vi "forceToVoltage.vi"(8 "error in (no error)":errorcluster, 9 "Pressure Servo Settings":T1={"Center Point"=2.5, "Area"=0.004536, "PA to PSI"=0.000145038, "Off Value"=0.004536} {"Off Value" format="%.3f"; "PA to PSI" format="%.9f"; "Area" format="%.9f"; "Center Point" format="%.3f"}, 10 "Force":dbl[unit], 11 "Force To Pressure Servo Valve Voltage in":refnum<class "Force To Pressure Servo Valve Voltage.lvclass">) -> (0 "error out":errorcluster, 1 "Voltage 2":dbl[unit], 2 "Voltage 1":dbl[unit], 3 "Force To Pressure Servo Valve Voltage out":refnum<class "Force To Pressure Servo Valve Voltage.lvclass">)   [LabVIEW 2015, in "Force To Pressure Servo Valve Voltage.lvclass"]
uses:
  Force To Pressure Servo Valve Voltage.lvclass
  Typedefs/Pressure Servo Valve Settings.ctl
  Typedefs/FAMT Typedefs.lvlib
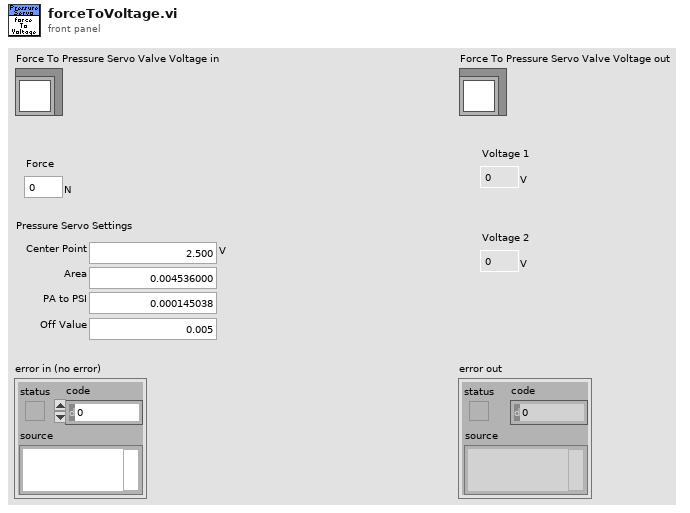
[diagram p1: front panel]
types:
  T1 = typedef "FAMT Typedefs.lvlib/Pressure Servo Valve Settings.ctl" = cluster{"Center Point":dbl[unit], "Area":dbl, "PA to PSI":dbl, "Off Value":dbl}
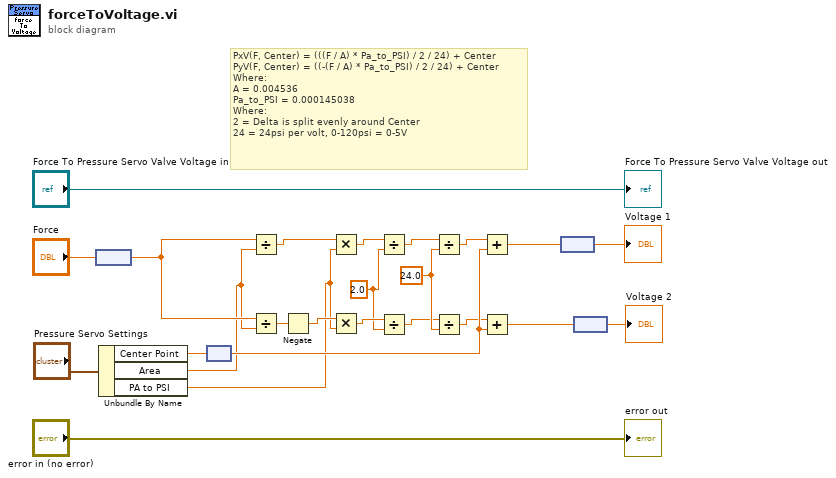
[diagram p0: block diagram]
diagram:
  w15 = 24.0 ("y")
  w19 = 2.0 ("y")
  # "PxV(F, Center) = (((F / A) * Pa_to_PSI) / 2 / 24) + Center\nPyV(F, Center) = ((-(F / A) * Pa_to_PSI) / 2 / 24) + Center\nWhere:\nA = 0.004536\nPa_to_PSI = 0.000145038\nWhere:\n2 = Delta is split evenly around Center\n24 = 24psi per volt, 0-120psi = 0-5V"
  n1 = node("Force") -> (w17:dbl)
  n2 = Unbundle By Name("Pressure Servo Settings") -> ("Center Point"=w9:dbl[unit], "Area"=w2:dbl, "PA to PSI"=w1:dbl)
  n3 = node(w9) -> (w16:dbl)
  n4 = Divide(x=w17, y=w2) -> (x/y=w22:dbl)
  n5 = Divide(x=w17, y=w2) -> (x/y=w24:dbl)
  n6 = Negate(x=w24) -> (-x=w23:dbl)
  n7 = Multiply(x=w22, y=w1) -> (x*y=w21:dbl)
  n8 = Multiply(x=w23, y=w1) -> (x*y=w20:dbl)
  n9 = Divide(x=w21, y=w19) -> (x/y=w7:dbl)
  n10 = Divide(x=w20, y=w19) -> (x/y=w8:dbl)
  n11 = Divide(x=w7, y=w15) -> (x/y=w6:dbl)
  n12 = Divide(x=w8, y=w15) -> (x/y=w5:dbl)
  n13 = Add(x=w6, y=w16) -> (x+y=w3:dbl)
  n14 = Add(x=w5, y=w16) -> (x+y=w4:dbl)
  n15 = node(w3) -> (→"Voltage 1":dbl[unit])
  n16 = node(w4) -> (→"Voltage 2":dbl[unit])
  "error out" <- "error in (no error)"
  "Force To Pressure Servo Valve Voltage out" <- "Force To Pressure Servo Valve Voltage in"
